vi "Add Frame Polygon.vi"(8 "error in (no error)":errorcluster, 10 "Point Array":T1[](array[typedef])=[{"Longitude"=0.0, "Latitude"=0.0}] {"Latitude" format="%#_10g"; "Longitude" format="%#_10g"}) -> (0 "error out":errorcluster)   [LabVIEW 2014]
uses:
  Lat Long Conversion/Controls/PointLatLon.ctl
  System.Drawing
  C:/Robotic Systems/Products/AgFalcon/Software/Ground Station/Data/Mapping DLL/GMap.NET.WindowsForms.dll
  Data/Mapping DLL/GMap.NET.WindowsForms.dll
  Reference/SubVI/Main Map Control Refernce.vi
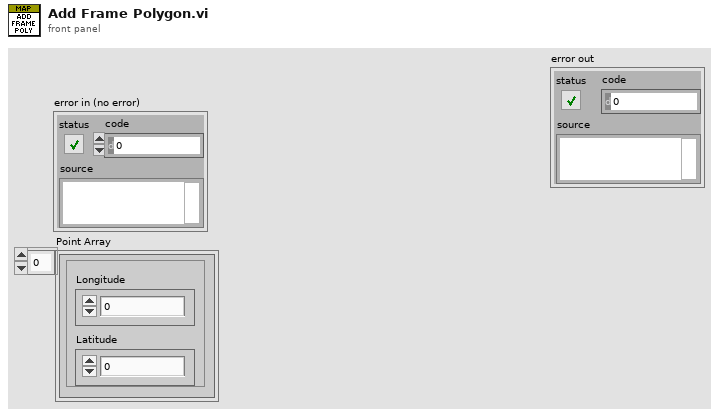
[diagram p1: front panel]
types:
  T1 = typedef "PointLatLon.ctl" = cluster{"Longitude":dbl, "Latitude":dbl}
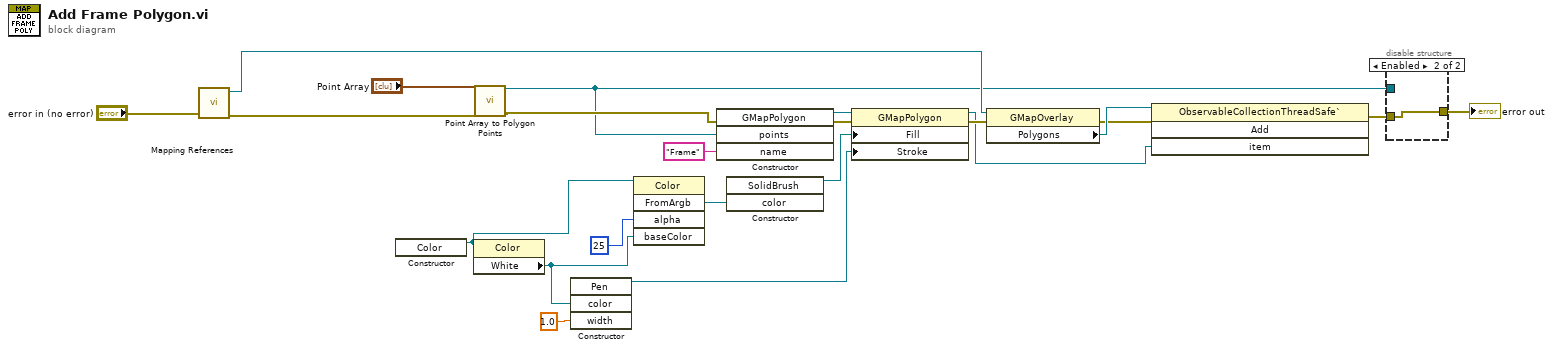
[diagram p0: block diagram]
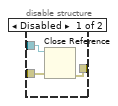
[diagram p2: hidden frame]
diagram:
  n1 = call-poly "Mapping References.vi"("Error In"="error in (no error)") -> ("Error Out"=w5:errorcluster, "Main Map Reference"=w4:refnum<k24>)  [unwired: 9 in]
  n2 = constructor class="Color"() -> (reference out=w14:refnum<k24>)  [unwired: 3 in, 2 out]
  n3 = property class="Color"(reference=w14) -> ("White"=w17:refnum<k24>)  [unwired: 1 in, 2 out]
  n4 = call "Point Array to Polygon Points.vi"("error in (no error)"=w5, "Point Array"="Point Array") -> ("error out"=w10:errorcluster, "Polygon Points"=w1:refnum<k24>)  [unwired: 8 in]
  n5 = constructor class="Pen"("color"=w17, "width"=sgl 1.0 ("Width")) -> (reference out=w16:refnum<k24>)  [unwired: 3 in, 4 out]
  n6 = invoke class="Color" method="FromArgb"(reference=w14, "alpha"=25, "baseColor"=w17) -> ("FromArgb"=w15:refnum<k24>)  [unwired: 2 in, 4 out]
  n7 = constructor class="GMapPolygon"(error in=w10, "points"=w1, "name"="Frame") -> (reference out=w21:refnum<k24>, error out=w20:errorcluster)  [unwired: 2 in, 3 out]
  n8 = constructor class="SolidBrush"("color"=w15) -> (reference out=w19:refnum<k24>)  [unwired: 3 in, 3 out]
  n9 = property class="GMapPolygon"(reference=w21, error in=w20, "Fill"=w19, "Stroke"=w16) -> (reference out=w11:refnum<k24>, error out=w13:errorcluster)
  n10 = property class="GMapOverlay"(reference=w4, error in=w13) -> (error out=w7:errorcluster, "Polygons"=w8:refnum<k24>)  [unwired: 1 out]
  n11 = invoke class="ObservableCollectionThreadSafe`" method="Add"(reference=w8, error in=w7, "item"=w11) -> (error out=w3:errorcluster)  [unwired: 1 in, 3 out]
  n12 = disable-structure shown="Enabled" {
    disable-tunnel: w3 -> [w25 w26]
    disable-tunnel: [w24 w26] -> w2
    disable-tunnel: w1 -> [w23 _]
    frame Disabled {
      n13 = Close Reference(reference=w23, error in (no error)=w25) -> (error out=w24:errorcluster)
    }
    frame Enabled {
    }
  }
  "error out" <- w2
